vi "PXI DAQ Engine.vi"() -> (2 "DAQ in Progress":bool)   [LabVIEW 2020]
doc: "Main thread controlling DAQ process. Waits on two notifiers from a higher-level measurement VI:\n\n<B>Start:</B> executes the main DAQ VI.\n\n<B>Abort:</B> terminates this thread, so that the higher-level VIs exit properly."
uses:
  Type Defs/PXI DAQ-Actions.ctl
  DAQ Engine VIs/PXI Globals.vi
panel:
  out "Notification":string
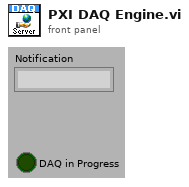
[diagram p1: front panel]
types:
  T1 = typedef "Semaphore RefNum" = refnum<k1>
  T2 = typedef "PXI DAQ-Actions.ctl" = enum16{"Set up", "Measure", "Trigger", "AO Queue", "Clean up"}
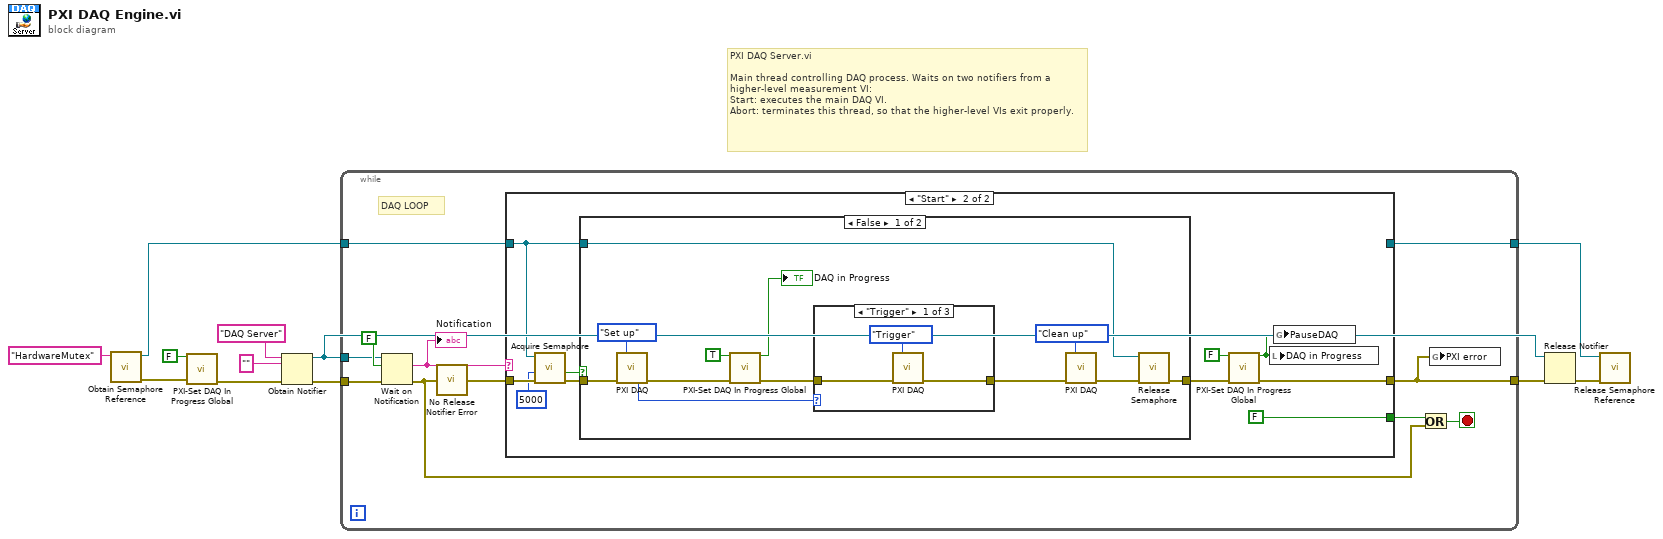
[diagram p0: block diagram]
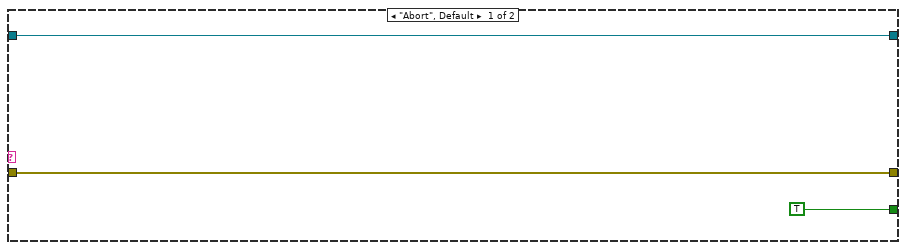
[diagram p2: hidden frame]
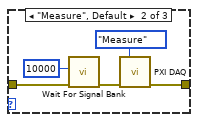
[diagram p3: hidden frame]
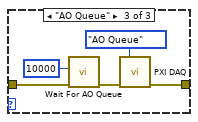
[diagram p4: hidden frame]
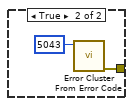
[diagram p5: hidden frame]
diagram:
  # "PXI DAQ Server.vi\n\nMain thread controlling DAQ process. Waits on two notifiers from a higher-level measurement VI:\nStart: executes the main DAQ VI.\nAbort: terminates this thread, so that the higher-level VIs exit properly."
  n1 = call <vilib>:"Obtain Semaphore Reference.vi"("name (unnamed)"="HardwareMutex") -> ("error out"=w5:errorcluster, "semaphore"=w3:T1)  [unwired: 4 in, 1 out]
  n2 = call "PXI-Set DAQ In Progress Global.vi"("In progress?"=FALSE, "error in (no error)"=w5) -> ("error out"=w7:errorcluster)  [unwired: 12 in, 1 out]
  n3 = Obtain Notifier(name (unnamed)="DAQ Server", notification data type="", error in (no error)=w7) -> (notifier out=w10:refnum<notifier>, error out=w11:errorcluster)  [unwired: 1 in, 1 out]
  n4 = while {
    tunnel: [w20] -> w9
    tunnel: w10 -> [w17]
    tunnel: w11 -> [w19]
    tunnel: w3 -> [w15]
    tunnel: [w14] -> w1
    stop <- w22 stop-if-true
    # "DAQ LOOP"
    n5 = Wait on Notification(notifier=w17, ignore previous (F)=FALSE, error in (no error)=w19) -> (notification=w16:string, error out=w13:errorcluster)  [unwired: 1 in, 2 out]
    "Notification" <- w16
    n6 = call "No Release Notifier Error.vi"("error in"=w13) -> ("error out"=w23:errorcluster)  [unwired: 14 in]
    n7 = case shown="\"Start\"" w16 {
      tunnel: w23 -> [w26 w35]
      tunnel: [w26 w33] -> w20
      tunnel: [TRUE FALSE] -> w18
      tunnel: w15 -> [w24 w29]
      tunnel: [w24 _] -> w14
      frame "Abort", Default {
      }
      frame "Start" {
        n8 = call <vilib>:"Acquire Semaphore.vi"("error in (no error)"=w35, "ms timeout (-1)"=5000, "semaphore"=w29) -> ("error out"=w31:errorcluster, "timed out"=w30:bool)  [unwired: 2 in, 1 out]
        n9 = case shown="False" w30 {
          tunnel: [w47 w63] -> w36
          tunnel: w31 -> [w48 _]
          tunnel: w29 -> [w46 _]
          frame False {
            n10 = call "PXI DAQ.vi"("Action"=PXI_DAQ-Actions."Set up", "error in (no error)"=w48) -> ("method"=w39:T2, "error out"=w45:errorcluster)  [unwired: 11 in, 1 out]
            n11 = call "PXI-Set DAQ In Progress Global.vi"("In progress?"=TRUE, "error in (no error)"=w45) -> ("In progress (out)"=→"DAQ in Progress":bool, "error out"=w43:errorcluster)  [unwired: 12 in]
            n12 = case shown="\"Trigger\"" w39 {
              tunnel: [w51 w56 w61] -> w44
              tunnel: w43 -> [w50 w54 w59]
              frame "Trigger" {
                n13 = call "PXI DAQ.vi"("Action"=PXI_DAQ-Actions."Trigger", "error in (no error)"=w50) -> ("error out"=w51:errorcluster)  [unwired: 11 in, 2 out]
              }
              frame "Measure", Default {
                n14 = call "Wait For Signal Bank.vi"("error in (no error)"=w54, "timeout (ms)"=10000) -> ("error out"=w55:errorcluster)  [unwired: 8 in, 1 out]
                n15 = call "PXI DAQ.vi"("Action"=PXI_DAQ-Actions."Measure", "error in (no error)"=w55) -> ("error out"=w56:errorcluster)  [unwired: 11 in, 2 out]
              }
              frame "AO Queue" {
                n16 = call "Wait For AO Queue.vi"("error in (no error)"=w59, "timeout (ms)"=10000) -> ("error out"=w60:errorcluster)  [unwired: 9 in]
                n17 = call "PXI DAQ.vi"("Action"=PXI_DAQ-Actions."AO Queue", "error in (no error)"=w60) -> ("error out"=w61:errorcluster)  [unwired: 11 in, 2 out]
              }
            }
            n18 = call "PXI DAQ.vi"("Action"=PXI_DAQ-Actions."Clean up", "error in (no error)"=w44) -> ("error out"=w40:errorcluster)  [unwired: 11 in, 2 out]
            n19 = call <vilib>:"Release Semaphore.vi"("error in (no error)"=w40, "semaphore"=w46) -> ("error out"=w47:errorcluster)  [unwired: 4 in, 1 out]
          }
          frame True {
            n20 = call <vilib>:"Error Cluster From Error Code.vi"("error code (0)"=5043) -> ("error out"=w63:errorcluster)  [unwired: 8 in]
          }
        }
        n21 = call "PXI-Set DAQ In Progress Global.vi"("In progress?"=FALSE, "error in (no error)"=w36) -> ("In progress (out)"=w27:bool, "error out"=w33:errorcluster)  [unwired: 12 in]
        n22 = local write "DAQ in Progress"(w27) -> ()
        n23 = global write "PXI Globals.vi" "PauseDAQ"(w27) -> ()
      }
    }
    n24 = Or(x=w18, y=w13) -> (x .or. y?=w22:bool)
    n25 = global write "PXI Globals.vi" "PXI error"(w20) -> ()
  }
  n26 = Release Notifier(notifier=w10, error in (no error)=w9) -> (error out=w2:errorcluster)  [unwired: 1 in, 2 out]
  n27 = call <vilib>:"Release Semaphore Reference.vi"("error in (no error)"=w2, "semaphore"=w1) -> ()  [unwired: 8 in, 2 out]
